vi "2 angle_iteration.vi"(1 "Phi":dbl, 2 "Apparent Wind\nSpeed":T1, 3 "Apparent Wind\nDirection (º)":T2) -> (0 "Best Theta":dbl)   [LabVIEW 2011]
doc: "Given one angle, this VI returns a partner angle which minimizes travel time to the waypoint. It does this by checking 180 different angles and returning the optimal one."
uses:
  2 Typedefs/apparent wind direction.ctl
  2 Typedefs/apparent wind speed.ctl
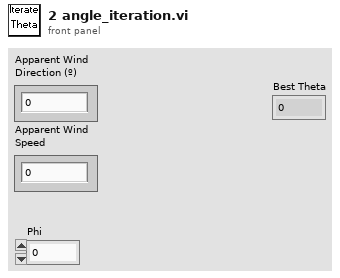
[diagram p1: front panel]
types:
  T1 = typedef "apparent wind speed.ctl" = dbl
  T2 = typedef "apparent wind direction.ctl" = dbl
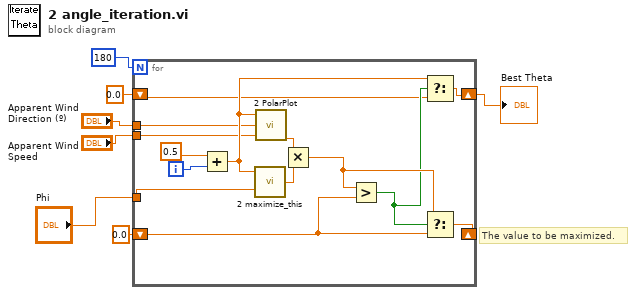
[diagram p0: block diagram]
diagram:
  # "The value to be maximized."
  n1 = for {
    N: 180 -> [_]
    tunnel: "Phi" -> [w19]
    shift-right: [w15] -> _
    shift-left: 0.0 -> [w14]
    shift-right: [w11] -> w3
    shift-left: 0.0 -> [w10]
    tunnel: "Apparent Wind\nDirection (º)" -> [w9]
    tunnel: "Apparent Wind\nSpeed" -> [w8]
    i -> [w21]
    n2 = Add(x=0.5, y=w21) -> (x+y=w12:dbl)
    n3 = call "2 maximize_this.vi"("Phi"=w19, "Theta"=w12) -> ("Value"=w17:dbl)  [unwired: 1 in]
    n4 = call "2 PolarPlot.vi"("Apparent Wind\nSpeed"=w8, "Apparent Wind\nDirection (º)"=w9, "Boat Angle"=w12) -> ("Velocity"=w18:dbl)
    n5 = Multiply(x=w18, y=w17) -> (x*y=w16:dbl)
    n6 = Greater?(x=w16, y=w14) -> (0:w13:bool)
    n7 = Select(t=w12, s=w13, f=w10) -> (s? t:f=w11:dbl)
    n8 = Select(t=w16, s=w13, f=w14) -> (s? t:f=w15:dbl)
  }
  "Best Theta" <- w3
